vi "Continuous Aquisition On.vi"(8 "error in":errorcluster, 9 "Acquition Speed":u32, 10 "Analog Input Pin":u8, 11 "Arduino Resource":T1={"VISA resource"="", "Board Type"=enum."Arduino Uno", "Connection Type"=enum."USB / Serial", "Bytes Per Packet (15)"=15}) -> (0 "error out":errorcluster, 3 "Arduino Resource":T1={"VISA resource"="", "Board Type"=enum."Arduino Uno", "Connection Type"=enum."USB / Serial", "Bytes Per Packet (15)"=15})   [LabVIEW 2011, in "LabVIEW Interface for ChipKit.lvlib"]
doc: "This VI puts the Arduino in continuous acquisition mode where it will continuously write analog samples to the serial port at the specified rate. The sample rate cannot be set to be faster than 5KHZ. While this mode is turned on executing other LIFA commands will corrupt analog data. To use other LIFA commands turn continuous mode off first."
uses:
  LabVIEW Interface for ChipKit.lvlib
  Private/Type Defs/Command.ctl
  Private/Type Defs/Board Type.ctl
  Private/Type Defs/Chipkit Resource.ctl
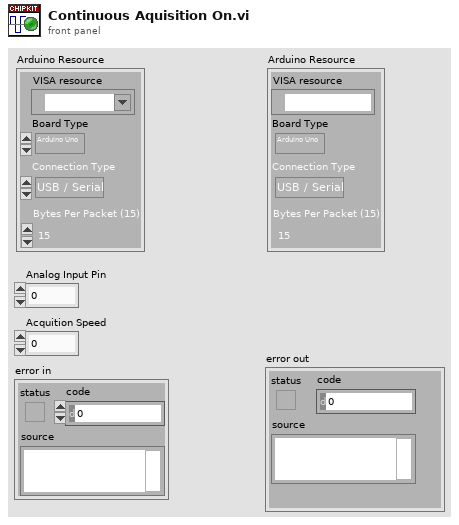
[diagram p1: front panel]
types:
  T1 = typedef "LabVIEW Interface for ChipKit.lvlib/Chipkit Resource.ctl" = cluster{"VISA resource":refnum<visa-resource-name>, "Board Type":T2, "Connection Type":enum8{"USB / Serial"}, "Bytes Per Packet (15)":u8}
  T2 = typedef "LabVIEW Interface for ChipKit.lvlib/Board Type.ctl" = enum16{"Arduino Uno", "Dimuelanove w/Atmega 328", "Mega 2560", "Chipkit Uno32", "Chipkit Max32"}
  T3 = typedef "LabVIEW Interface for ChipKit.lvlib/Command.ctl" = enum8{"setArduinoMode", "flushSerial", "setPinMode", "digitalWritePin", "digitalWritePort", "tone", "digitalReadPin", "digitalReadPort", "analogReadPin", "analogReadPort", "pwmWritePin", "pwmWritePort", "sevenSegment_Configure", "sevenSegment_Write", "I2C Init", "I2C Write", "I2C Read", "SPI Init", "SPI Set Bit Order", "SPI Set Clock Divider", "SPI Set Data Mode", "SPI Send / Receive", "SPI Close", "Servo Set Num Servos", "Servo Config Servo", "Servo Write Angle", "Servo Read Angle", "Servo Write Pulse Width", "Servo Read Pulse Width", "Servo Detach", "LCD Init", "LCD Set Size", "LCD Set Cursor Mode", "LCD Clear", "LCD Set Cursor Position", "LCD Print", "LCD Display Power", "LCD Scroll Display", "LCD Autoscroll", "LCD Print Direction", "LCD Create Custom Char", "LCD Print Custom Char", "contAcqOn", "contAcqOff", "getFirmwareVersion", "FiniteSampleStart"}
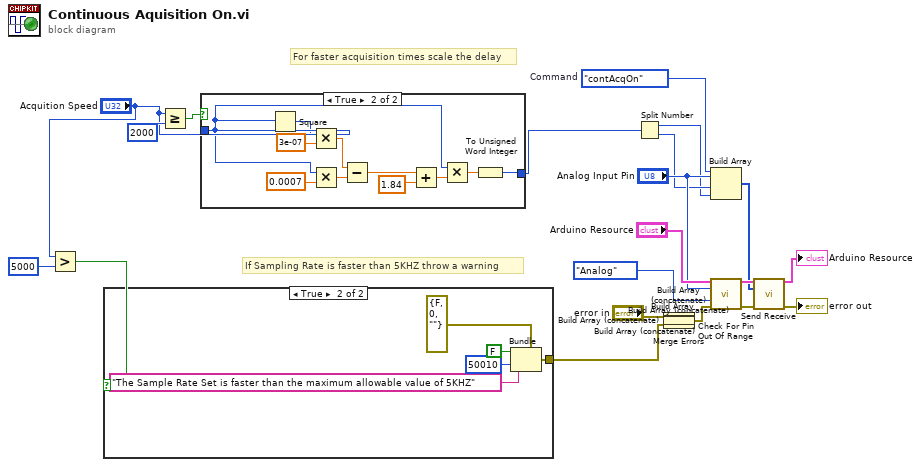
[diagram p0: block diagram]
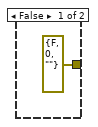
[diagram p2: hidden frame]
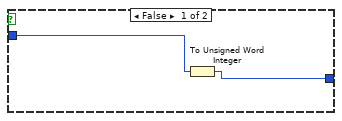
[diagram p3: hidden frame]
diagram:
  w22 = Command."contAcqOn"  # Command
  # "If Sampling Rate is faster than 5KHZ throw a warning"
  # "For faster acquisition times scale the delay"
  n1 = Greater?(x="Acquition Speed", y=u16 5000) -> (0:w11:bool)
  n2 = case shown="True" w11 {
    tunnel: [errorcluster {"status"=FALSE, "code"=0, "source"=""} ("error out") w27] -> w8
    frame False {
    }
    frame True {
      n3 = Bundle(cluster=errorcluster {"status"=FALSE, "code"=0, "source"=""} ("error out"), "status"=FALSE, "code"=50010, "source"="The Sample Rate Set is faster than the maximum allowable value of 5KHZ") -> (w27:errorcluster)
    }
  }
  n4 = Greater Or Equal?(x="Acquition Speed", y=2000) -> (x >= y?=w15:bool)
  n5 = case shown="True" w15 {
    tunnel: "Acquition Speed" -> [w32 w34]
    tunnel: [w33 w37] -> w13
    frame False {
      n6 = To Unsigned Word Integer(number=w32) -> (unsigned 16bit integer=w33:u16)
    }
    frame True {
      n7 = Square(x=w34) -> (x^2=w44:u32)
      n8 = Multiply(x=w44, y=3e-07) -> (x*y=w42:dbl)
      n9 = Multiply(x=w34, y=0.0007) -> (x*y=w41:dbl)
      n10 = Subtract(x=w42, y=w41) -> (x-y=w39:dbl)
      n11 = Add(x=w39, y=1.84) -> (x+y=w36:dbl)
      n12 = Multiply(x=w34, y=w36) -> (x*y=w35:dbl)
      n13 = To Unsigned Word Integer(number=w35) -> (unsigned 16bit integer=w37:u16)
    }
  }
  n14 = Split Number(x=w13) -> (hi(x)=w16:u8, lo(x)=w17:u8)
  n15 = Build Array("error in", w8) -> (w5:errorcluster[])
  n16 = Build Array (concatenate)(w5) -> (w4:errorcluster[])
  n17 = Build Array (concatenate)(w4) -> (w3:errorcluster[])
  n18 = Build Array (concatenate)(w3) -> (w2:errorcluster[])
  n19 = Build Array (concatenate)(w2) -> (w1:errorcluster[])
  n20 = Merge Errors(w1) -> (w6:errorcluster)
  n21 = Build Array(w22, "Analog Input Pin", w17, w16) -> (w20:u8[])
  n22 = call "Check For Pin Out Of Range.vi"("Arduino Resource"="Arduino Resource", "User Pin Number"="Analog Input Pin", "Pin Type"=enum16{"Analog", "Digital"}."Analog", "error in"=w6) -> ("Arduino Resource"=w23:T1, "error out"=w24:errorcluster)  [unwired: 10 in]
  n23 = call "Send Receive.vi"("Arduino Resource"=w23, "Data"=w20, "error in"=w24) -> ("Arduino Resource"=→"Arduino Resource":T1, "error out"=→"error out":errorcluster)  [unwired: 10 in, 1 out]
